vi "BoneIP_Init.vi"(2 "error in":errorcluster, 3 "Task":enum16{"Init", "Close"}(ring), 4 "Connection in":T1) -> (0 "error out":errorcluster, 1 "Connection Out":T1)   [LabVIEW 2012]
uses:
  <userlib>/BotSpeak/VIs/SubVIs/CommState.ctl
  <userlib>/BotSpeak/VIs/Direct/BotSpeak_Control.ctl
panel:
  out "String":string
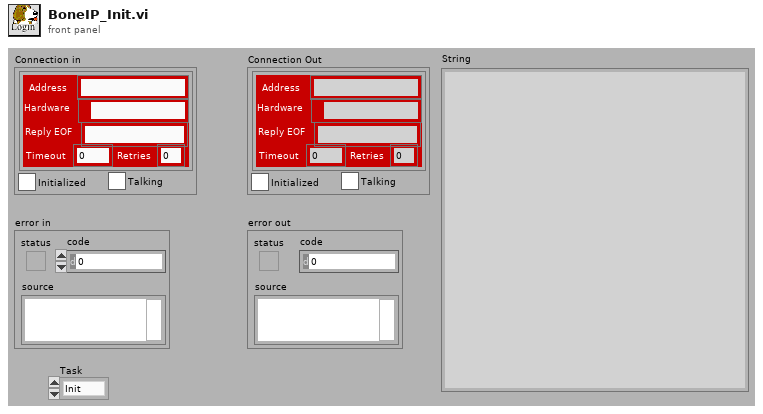
[diagram p1: front panel]
types:
  T1 = typedef "CommState.ctl" = cluster{"Bot Settings":T2, "Initialized":bool, "Talking":bool}
  T2 = typedef "BotSpeak_Control.ctl" = cluster{"Address":string, "Reply EOF":string, "Hardware":path, "Retries":i8, "Timeout":i32}
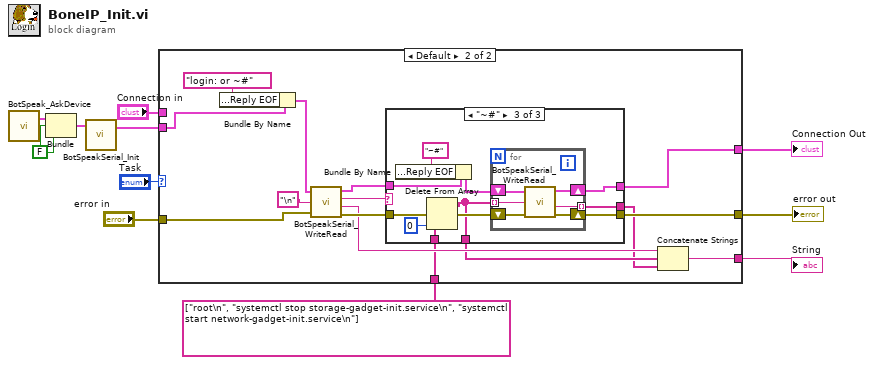
[diagram p0: block diagram]
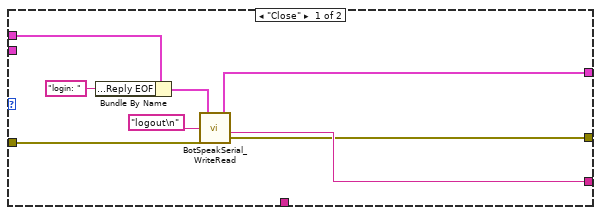
[diagram p2: hidden frame]
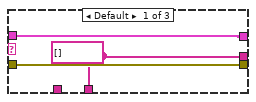
[diagram p3: hidden frame]
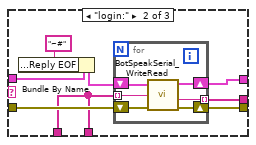
[diagram p4: hidden frame]
diagram:
  w3 = FALSE
  n1 = call <userlib>:"BotSpeak_AskDevice.vi"() -> ("Bot Settings out"=w4:T2)  [unwired: 3 in]
  n2 = Bundle("Bot Settings out"=w4, w3, w3) -> (w2:cluster{"Bot Settings out":T2, bool, bool})  [unwired: 1 in]
  n3 = call <userlib>:"BotSpeakSerial_Init.vi"("Connection In"=w2) -> ("Connection out"=w1:T1)  [unwired: 1 in, 1 out]
  n4 = case shown="Default" "Task" {
    tunnel: [w17 w34] -> w11
    tunnel: [w15 w32] -> w10
    tunnel: "Connection in" -> [w14 _]
    tunnel: [w18 w24] -> w8
    tunnel: "error in" -> [w16 w22]
    tunnel: string[] ["root\n", "systemctl stop storage-gadget-init.service\n", "systemctl start network-gadget-init.service\n"] -> [_ w21]
    tunnel: w1 -> [_ w20]
    frame "Close" {
      n5 = Bundle By Name(cluster=w14, "Bot Settings.Reply EOF"="login: ") -> (w13:T1)
      n6 = call <userlib>:"BotSpeakSerial_WriteRead.vi"("error In"=w16, "To Write"="logout\n" ("String To Send"), "Connection In"=w13) -> ("error out"=w17:errorcluster, "Reply"=w18:string, "Connection Out"=w15:T1)  [unwired: 1 out]
    }
    frame Default {
      n7 = Bundle By Name(cluster=w20, "Bot Settings.Reply EOF"="login: or ~#" ("Status String")) -> (w29:T1)
      n8 = call <userlib>:"BotSpeakSerial_WriteRead.vi"("error In"=w22, "To Write"="\n" ("Status String"), "Connection In"=w29) -> ("error out"=w33:errorcluster, "Reply"=w27:string, "Reply EOF"=w23:string, "Connection Out"=w31:T1)
      n9 = case shown="\"~#\"" w23 {
        tunnel: [w36 w45 w61] -> w34
        tunnel: w33 -> [w36 w44 w60]
        tunnel: [w37 w43 w59] -> w32
        tunnel: w31 -> [w37 w40 w56]
        tunnel: [w35 w38 w53] -> w26
        tunnel: [w35 w39 w55] -> w25
        tunnel: w21 -> [_ w38 w54]
        frame Default {
          w35 = string[] []
        }
        frame "login:" {
          n10 = Bundle By Name(cluster=w40, "Bot Settings.Reply EOF"="~#" ("Status String")) -> (w42:T1)
          n11 = for {
            tunnel: w38 -> [w47] mode=indexing
            tunnel: [w46] -> w39 mode=indexing
            shift-right: [w49] -> w43
            shift-left: w42 -> [w48]
            shift-right: [w51] -> w45
            shift-left: w44 -> [w50]
            n12 = call <userlib>:"BotSpeakSerial_WriteRead.vi"("error In"=w50, "To Write"=w47, "Connection In"=w48) -> ("error out"=w51:errorcluster, "Reply"=w46:string, "Connection Out"=w49:T1)  [unwired: 1 out]
          }
        }
        frame "~#" {
          n13 = Bundle By Name(cluster=w56, "Bot Settings.Reply EOF"="~#" ("Status String")) -> (w58:T1)
          n14 = Delete From Array(array=w54, index=0) -> (array with subset deleted=w53:string[])  [unwired: 1 in, 1 out]
          n15 = for {
            tunnel: [w63] -> w55 mode=indexing
            shift-right: [w65] -> w59
            shift-left: w58 -> [w64]
            shift-right: [w67] -> w61
            shift-left: w60 -> [w66]
            tunnel: w53 -> [w62] mode=indexing
            n16 = call <userlib>:"BotSpeakSerial_WriteRead.vi"("error In"=w66, "To Write"=w62, "Connection In"=w64) -> ("error out"=w67:errorcluster, "Reply"=w63:string, "Connection Out"=w65:T1)  [unwired: 1 out]
          }
        }
      }
      n17 = Concatenate Strings(w27, w26, w25) -> (w24:string)
    }
  }
  "error out" <- w11
  "Connection Out" <- w10
  "String" <- w8
